vi "Max_And_Min_Speed.vi"(10 "Time Array":dbl[](array[numeric]), 11 "Linear Speed Array":dbl[](array[numeric])) -> (3 "Min/Max Linear Speed":T1 {"Maximum Linear Speed (m/s)" format="%#_3g"})   [LabVIEW 2018]
doc: "This VI finds the values of maximum and minimum linear speed and the time at which it occurred. It does so by using the 'Array Max & Min' function, thus finding the maximum and minimum values and the indexes of these values. The time values of these events are found using the previously mentioned indexes using 'Index Array' function. This data is then bundled into two 'clusters of 2 elements'.\n\nInputs:\nChange in linear speed array;\nTime array.\n\nOutputs:\nMin/Max Linear Speed."
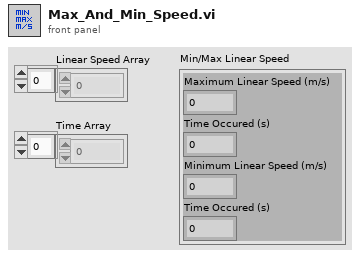
[diagram p1: front panel]
types:
  T1 = cluster{"Maximum Linear Speed (m/s)":dbl, "Time Occured (s)":dbl, "Minimum Linear Speed (m/s)":dbl, "Time Occured (s)":dbl}
  T2 = cluster{dbl, "Current Time (s)":dbl, dbl, "Current Time (s)":dbl}
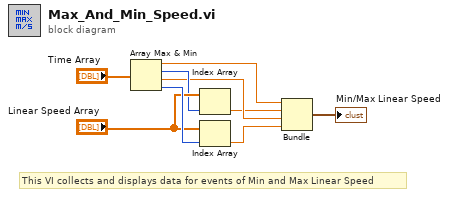
[diagram p0: block diagram]
diagram:
  # "This VI collects and displays data for events of Min and Max Linear Speed"
  n1 = Array Max & Min(array="Time Array") -> (max value=w5:dbl, max index (indices)=w7:i32, min value=w4:dbl, min index (indices)=w9:i32)
  n2 = Index Array(array="Linear Speed Array", index=w7) -> (element=w3:dbl)
  n3 = Index Array(array="Linear Speed Array", index=w9) -> (element=w2:dbl)
  n4 = Bundle(w5, "Current Time (s)"=w3, w4, "Current Time (s)"=w2) -> (→"Min/Max Linear Speed":T2)  [unwired: 1 in]
